vi "NormalAttackerRoleVSS.vi"(7 "First call?":bool=TRUE, 8 "error in (no error)":errorcluster, 9 "Game in":refnum<class "Game.lvclass">, 10 "Robot":refnum<class "Robot.lvclass">, 11 "NormalAttackerRoleVSS in":refnum<class "NormalAttackerRoleVSS.lvclass">) -> (0 "error out":errorcluster, 1 "Game out":refnum<class "Game.lvclass">, 2 "Robot out":refnum<class "Robot.lvclass">, 3 "NormalAttackerRoleVSS out":refnum<class "NormalAttackerRoleVSS.lvclass">)   [LabVIEW 2020, in "NormalAttackerRoleVSS.lvclass"]
uses:
  NormalAttackerRoleVSS.lvclass
  C:/Users/lucio/Desktop/Horie/ROBOIME/VSS_AI/Role_class/Role.lvclass
  Robot_class/Robot.lvclass
  Game_class/Game.lvclass
  Role_class/Role.lvclass/Role.ctl
  Role_class/Read Tacticbook.vi
  Role_class/Write Tacticbook.vi
  Tacticbook_class/Tacticbook.lvclass
  DispBallTacticVSS_class/DispBallTacticVSS.lvclass
  DefendGoalTacticVSS_class/DefendGoalTacticVSS.lvclass
  PenaltyAttackTacticVSS_class/PenaltyAttackTacticVSS.lvclass
  DefendAreaTacticVSS_class/DefendAreaTacticVSS.lvclass
  AttackTacticVSS_class/AttackTacticVSS.lvclass
  HaltTactic_class/HaltTactic.lvclass
  GoAndKickTacticVSS_class/GoAndKickTacticVSS.lvclass
  GoalKickKeeperTacticVSS_class/GoalKickKeeperTacticVSS.lvclass
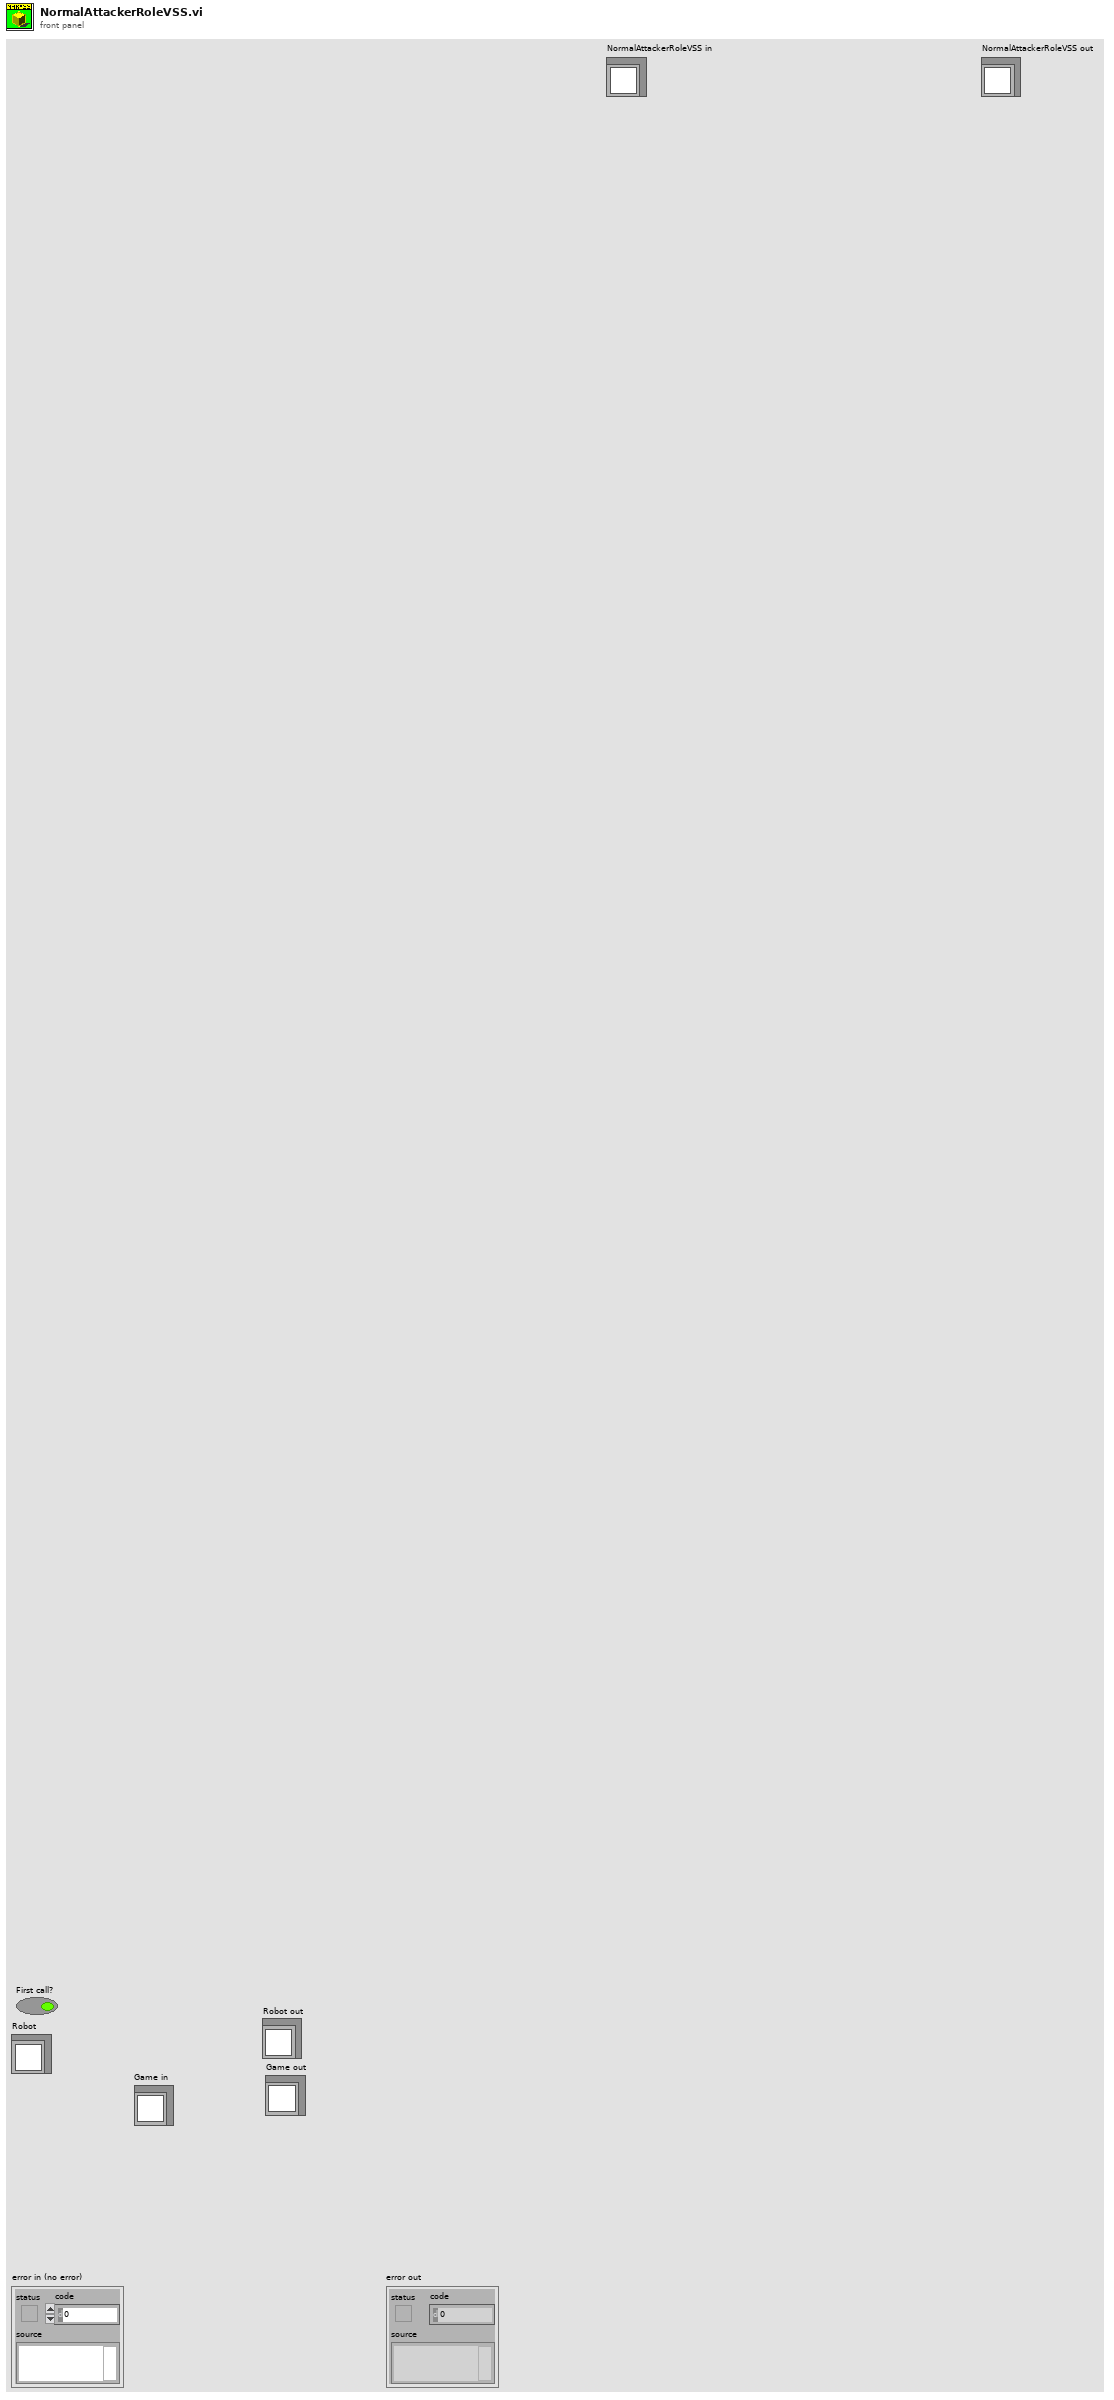
[diagram p1: front panel]
types:
  T1 = enum16{"AttackTacticVSS", "CounterAttackTacticVSS", "Exit"}
  T2 = cluster{"DispBallTacticVSS":refnum<class "DispBallTacticVSS.lvclass">, "DefendGoalTacticVSS":refnum<class "DefendGoalTacticVSS.lvclass">, "PenaltyAttackTacticVSS":refnum<class "PenaltyAttackTacticVSS.lvclass">, "DefendAreaTacticVSS":refnum<class "DefendAreaTacticVSS.lvclass">, "AttackTacticVSS":refnum<class "AttackTacticVSS.lvclass">, "HaltTactic":refnum<class "HaltTactic.lvclass">, "GoAndKickTacticVSS":refnum<class "GoAndKickTacticVSS.lvclass">, "GoalKickKeeperTacticVSS":refnum<class "GoalKickKeeperTacticVSS.lvclass">}
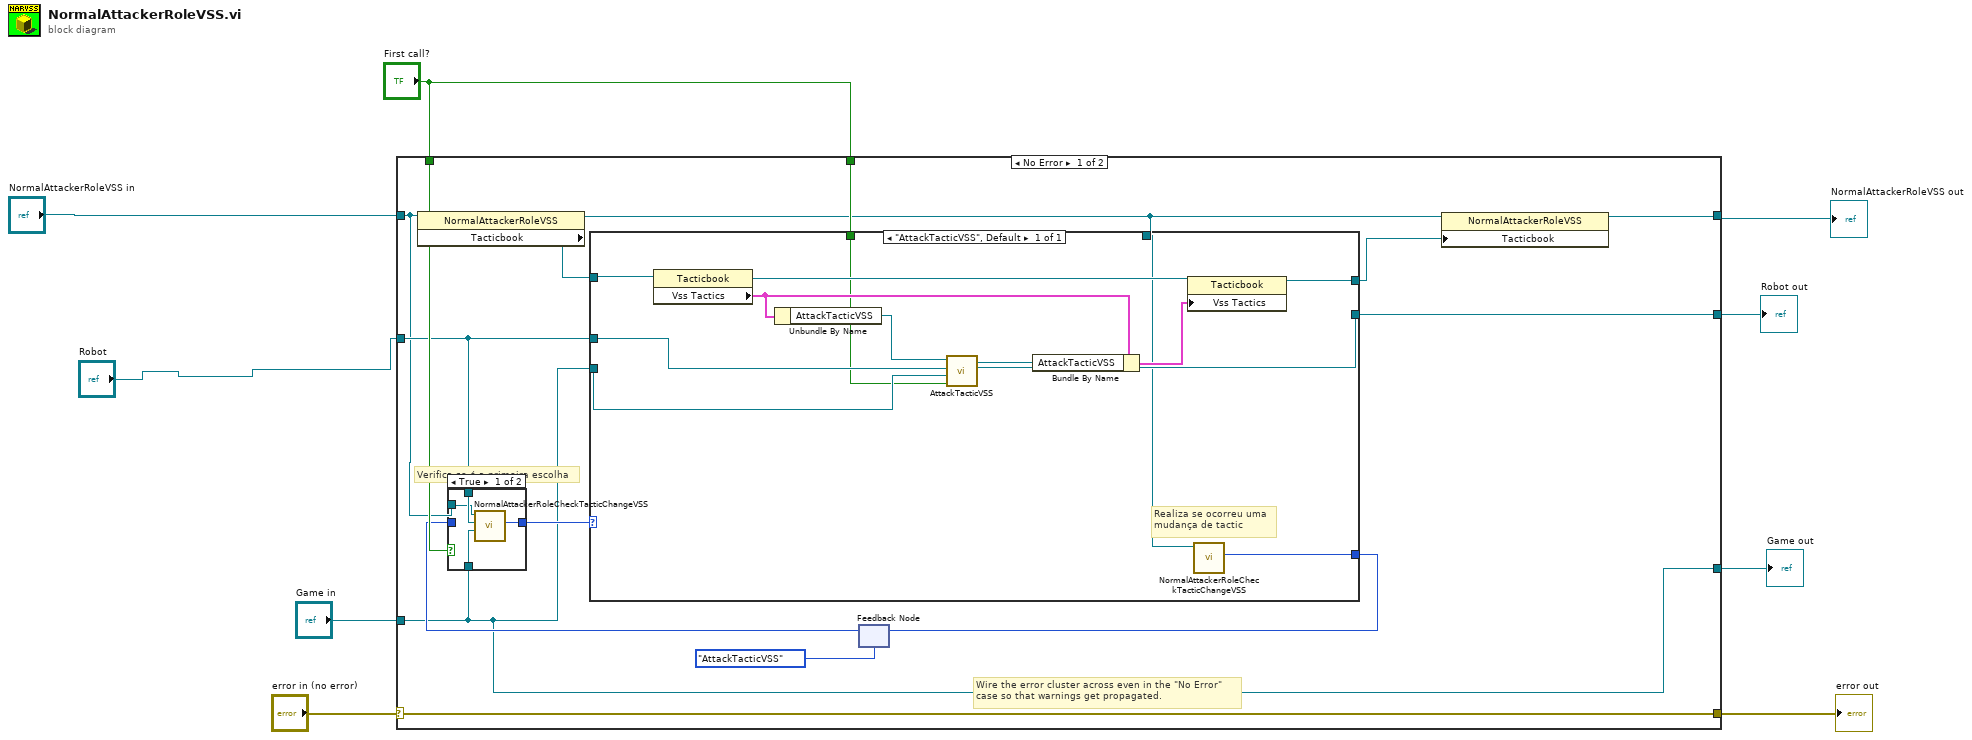
[diagram p0: block diagram]
diagram:
  n1 = case shown="No Error" "error in (no error)" {
    selector: "error in (no error)" -> [w24 w46]
    tunnel: [w24 w46] -> w8
    tunnel: [w23 w45] -> w3
    tunnel: "NormalAttackerRoleVSS in" -> [w11 w45]
    tunnel: "Robot" -> [w12 w44]
    tunnel: [w21 w44] -> w7
    tunnel: [w13 w43] -> w6
    tunnel: "Game in" -> [w13 w43]
    tunnel: "First call?" -> [w19 _]
    tunnel: "First call?" -> [w18 _]
    frame No Error {
      # "Verifica se é a primeira escolha"
      # "Wire the error cluster across even in the \"No Error\"\ncase so that warnings get propagated."
      n2 = property class="NormalAttackerRoleVSS"(reference=w11) -> (reference out=w10:refnum<class "NormalAttackerRoleVSS.lvclass">, "Tacticbook"=w22:refnum<class "Tacticbook.lvclass">)  [unwired: 1 in, 1 out]
      n3 = feedback #1(T1."AttackTacticVSS" ("Tactic")) -> (w17:T1)
      n4 = case shown="True" w18 {
        tunnel: w17 -> [_ w29]
        tunnel: [w28 w29] -> w16
        tunnel: w13 -> [w27 _]
        tunnel: w12 -> [w26 _]
        tunnel: w11 -> [w25 _]
        frame True {
          n5 = call "NormalAttackerRoleCheckTacticChangeVSS.vi"("Game in"=w27, "Robot In"=w26, "NormalAttackerRoleVSS in"=w25) -> ("Tactic"=w28:T1)  [unwired: 6 in, 2 out]
        }
        frame False {
        }
      }
      n6 = case shown="\"AttackTacticVSS\", Default" w16 {
        tunnel: w22 -> [w42]
        tunnel: w12 -> [w36]
        tunnel: [w34] -> w21
        tunnel: [w40] -> w20
        tunnel: w13 -> [w35]
        tunnel: w19 -> [w33]
        tunnel: [w31] -> w14
        tunnel: w10 -> [w30]
        frame "AttackTacticVSS", Default {
          # "Realiza se ocorreu uma\nmudança de tactic"
          n7 = property class="Tacticbook"(reference=w42) -> (reference out=w41:refnum<class "Tacticbook.lvclass">, "Vss Tactics"=w39:T2)  [unwired: 1 in, 1 out]
          n8 = Unbundle By Name(w39) -> ("AttackTacticVSS"=w37:refnum<class "AttackTacticVSS.lvclass">)
          n9 = call "AttackTacticVSS.vi"("First call?"=w33, "Game in"=w35, "Robot"=w36, "AttackTacticVSS in"=w37) -> ("Robot out"=w34:refnum<class "Robot.lvclass">, "AttackTacticVSS out"=w32:refnum<class "AttackTacticVSS.lvclass">)  [unwired: 5 in, 1 out]
          n10 = Bundle By Name(cluster=w39, "AttackTacticVSS"=w32) -> (w38:T2)
          n11 = property class="Tacticbook"(reference=w41, "Vss Tactics"=w38) -> (reference out=w40:refnum<class "Tacticbook.lvclass">)  [unwired: 1 in, 1 out]
          n12 = call "NormalAttackerRoleCheckTacticChangeVSS.vi"("NormalAttackerRoleVSS in"=w30) -> ("Tactic"=w31:T1)  [unwired: 8 in, 2 out]
        }
      }
      n13 = feedback-in #1(w14) -> ()
      n14 = property class="NormalAttackerRoleVSS"(reference=w10, "Tacticbook"=w20) -> (reference out=w23:refnum<class "NormalAttackerRoleVSS.lvclass">)  [unwired: 1 in, 1 out]
    }
    frame Error {
    }
  }
  "NormalAttackerRoleVSS out" <- w3
  "error out" <- w8
  "Robot out" <- w7
  "Game out" <- w6
